vi "CommonVIs_UpdateClassMethods.vi"(1 "ClassPath/LvClassRef":variant, 2 "Methods":string[](array[string]), 4 "AllowPropertyMethod(True)":bool=TRUE, 5 "error in (no error)":errorcluster, 6 "BaseClass":bool, 7 "Don'tShowDialog(False)":bool, 8 "UseVirtualMethods(True)":bool=TRUE) -> (19 "error out":errorcluster)   [LabVIEW 2020]
uses:
  <resource>/Framework/Providers/Open_GDS/ClassProviders/Provider_LvNativeClass/ClassWriterNative_class/ClassWriterNative.lvclass
  <resource>/Framework/Providers/Open_GDS/ClassProviders/Provider_BaseClassInterface/CreateMethodData.ctl
  <resource>/Framework/Providers/Open_GDS/ClassProviders/Provider_EndevoGOOP300/GOOP300_SubVIs/GOOP300_MethodScopeType.ctl
  <resource>/Framework/Providers/Open_GDS/ClassProviders/Provider_LvNativeClass/ClassWriterNative_class/IconDetails.ctl
  <resource>/Framework/Providers/Open_GDS/ClassProviders/Provider_LvNativeClass/ClassWriterNative_class/IconSize.ctl
  <resource>/Framework/Providers/Open_GDS/ClassProviders/Provider_BaseClassInterface/ClassReader_class/ClassReader.lvclass
  <resource>/Framework/Providers/Open_GDS/ClassProviders/Provider_BaseClassInterface/ClassWriter_class/ClassWriter.lvclass
panel:
  out "Creating methods":u8(slide) scale=0.0..100.0
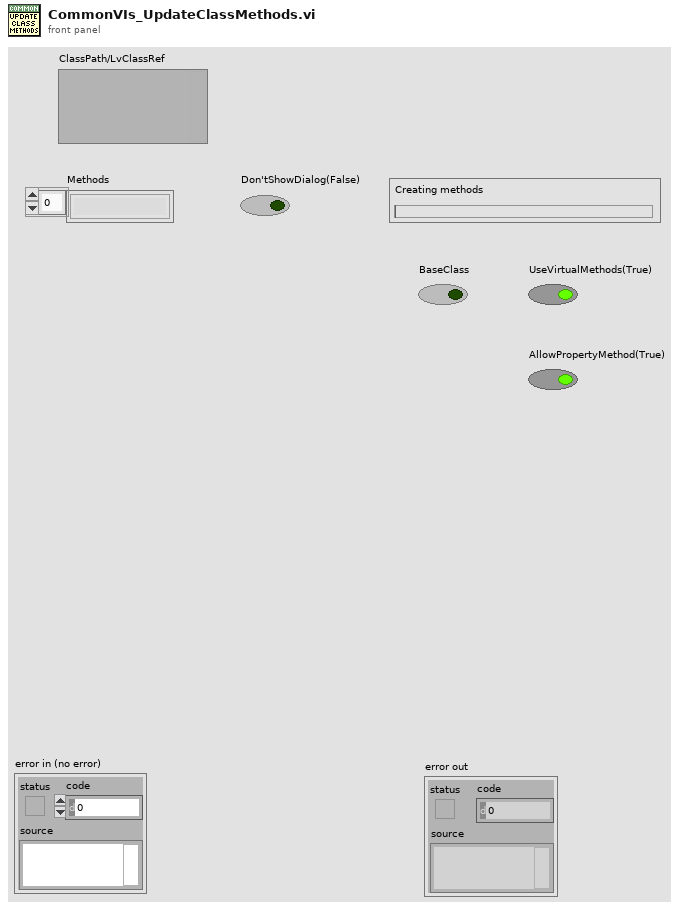
[diagram p1: front panel]
types:
  T1 = cluster{"Methods":cluster{"MethodName":string, "Private":bool, "Virtual":bool, "Reentrant":bool, "Description":string, "Icon Method Name":string, "Protected":bool, "Method Type":enum16{"Get", "Set", "GetProperty", "SetProperty"}, "Attribute":string, "ClassAtt":bool}[], "MethodPaths":path[], "MethodPrivate":bool[], "ClassItemRef":refnum<vi>}
  T2 = cluster{"MethodName":string, "Private":bool, "Virtual":bool, "Reentrant":bool, "Description":string, "Icon Method Name":string, "Protected":bool, "Method Type":enum16{"Get", "Set", "GetProperty", "SetProperty"}, "Attribute":string, "ClassAtt":bool}
  T3 = cluster{"MethodName":string, "Private":bool, "Virtual":bool, "Reentrant":bool, "Description":string, "Icon Method Name":string, "Protected":bool, "Method Type":enum16{"Get", "Set", "GetProperty", "SetProperty"}, "Attribute":string, "ClassAtt":bool}[]
  T4 = enum16{"Get", "Set", "GetProperty", "SetProperty"}
  T5 = typedef "ClassWriter.lvclass/CreateMethodData.ctl" = cluster{"MethodName":string, "RelativeMethodPath":path, "MethodDescription":string, "Scope/Visibility":T6, "MethodTemplateName":string, "IconOut":u8[][], "RelativeProjectClassPath":string, "OpenViAfterCreation":bool, "DynamicDispatchVi":bool, "ExtraCreateParameters":variant, "MustOverride":bool, "MustCallParent":bool, "IconDetails":T7, "AF-Option":variant, "TemplatePath":path}
  T6 = typedef "GOOP300_MethodScopeType.ctl" = enum16{"Use Parent Folder Scope", "Public", "Protected", "Private", "Community"}
  T7 = typedef "ClassWriterNative.lvclass/IconDetails.ctl" = cluster{"IconSize":T8, "ImageRows(32)":i32, "ConnectorPaneHeight":i32[]}
  T8 = typedef "ClassWriterNative.lvclass/IconSize.ctl" = enum16{"Full", "1 c-term high", "2 c-term high", "3 c-term high"}
  T9 = cluster{"AttributeNames":string[], "PropertyNode":bool, "FolderNames":string[]}
  T10 = typedef "ClassTypes_MethodType.ctl" = cluster{"MethodName":string, "Visibility":enum16{"Public", "Private", "Protected"}, "StereoType":string, "Path":path}
  T11 = typedef "CommonVIs_AttributeInfoType.ctl" = cluster{"name":string, "type":T12, "dimension":i32, "typeName":string, "typePath":path, "visibility":T13}
  T12 = typedef "CommonVIs_AttributeDataType.ctl" = enum16{"UINT8", "INT8", "UINT16", "INT16", "UINT32", "INT32", "UINT64", "INT64", "SGL", "DBL", "EXT", "CSG", "CDB", "CXT", "TimeStamp", "STRING", "PATH", "BOOL", "ENUM", "RefNum", "VIRefNum", "LabVIEW Class", "Cluster", "Variant", "TypeDef", "Waveform", "LabVIEW Object", "Other", "void", "Set", "Map"}
  T13 = typedef "CommonVIs_VisibilityType.ctl" = enum16{"Public", "Private", "Protected"}
  T14 = typedef "GDSLvCLass_ClassSettingsType.ctl" = cluster{"ClassProviderName":string, "ClassTemplateUsed":string, "ClassTemplateVersion":string, "ClassDescription":string, "PlugIns":T15[], "ConnectorPanePattern":string}
  T15 = typedef "GDSLvClass_PlugIn.ctl" = cluster{"Type":T16, "ID":string, "Version":string, "Path":path, "Name":string, "Data":variant}
  T16 = typedef "GDSLvClass_PlugInTypes.ctl" = enum16{"DesignPattern", "MethodTypes"}
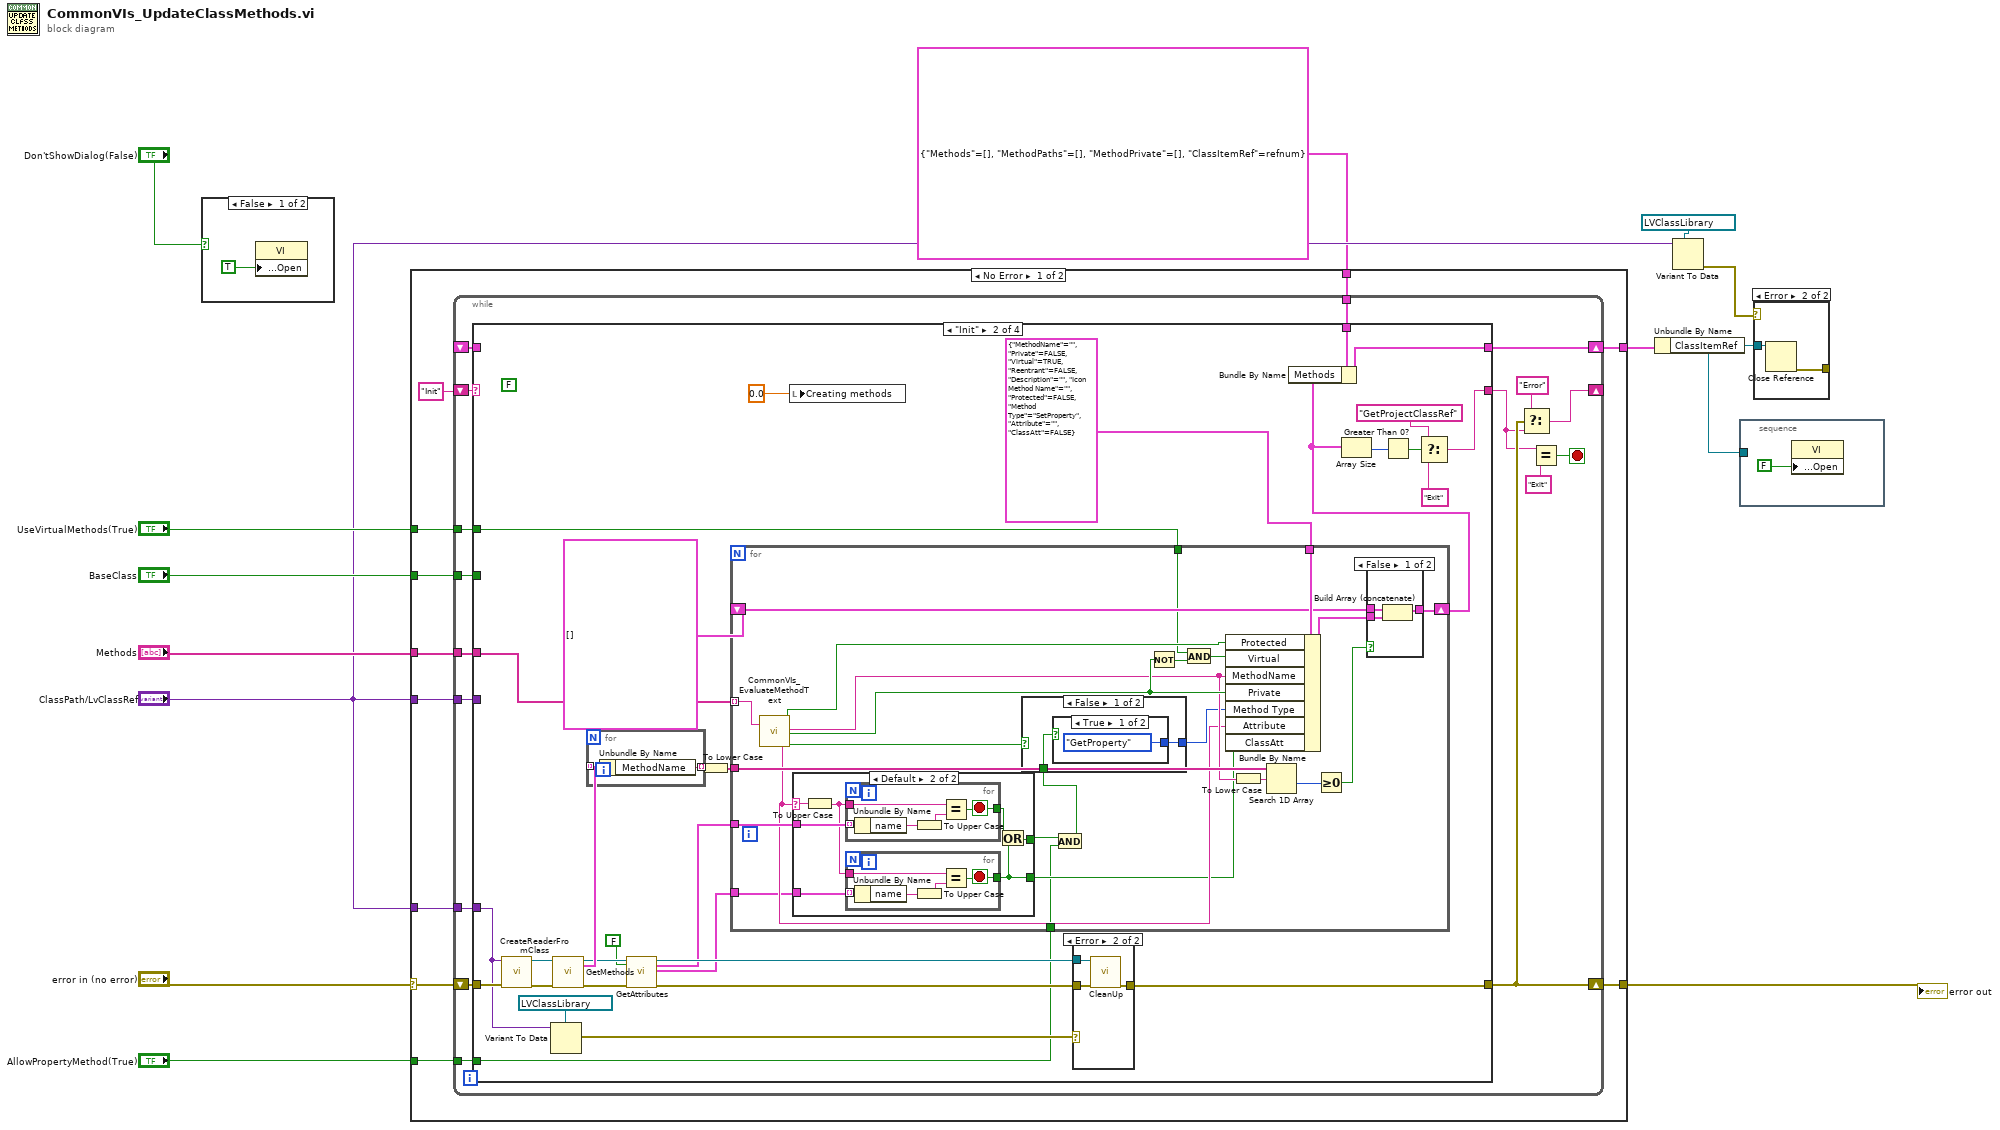
[diagram p0: block diagram]
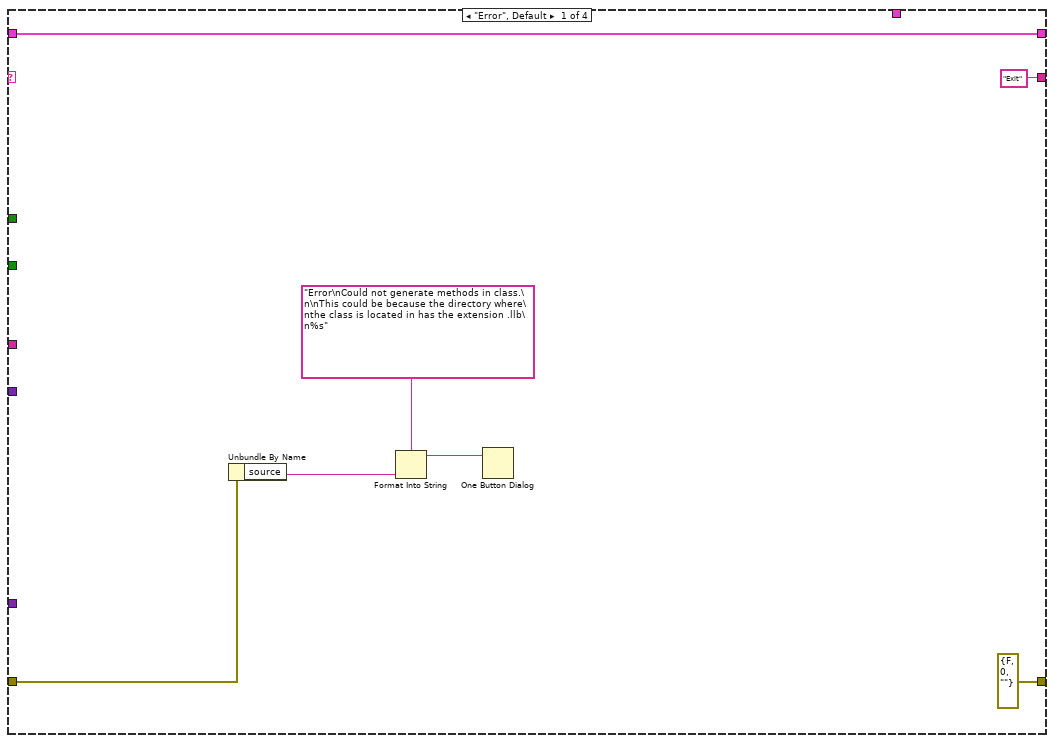
[diagram p4: hidden frame]
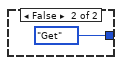
[diagram p7: hidden frame]
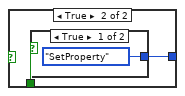
[diagram p8: hidden frame]
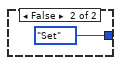
[diagram p9: hidden frame]
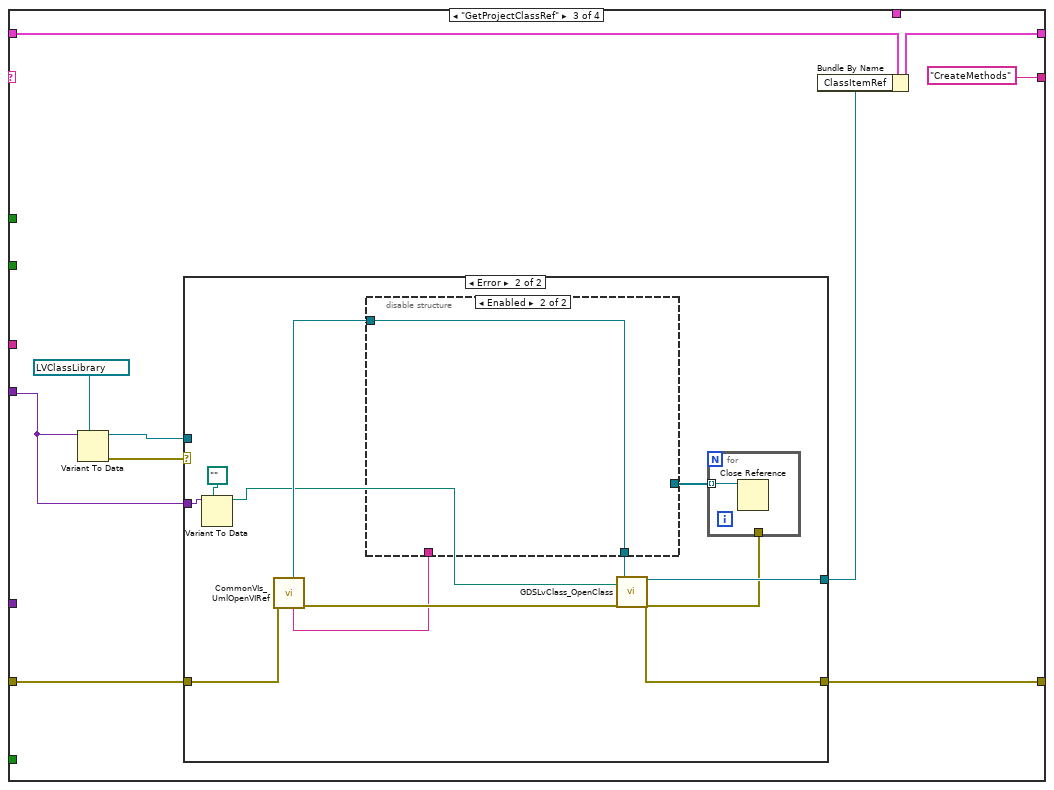
[diagram p11: hidden frame]
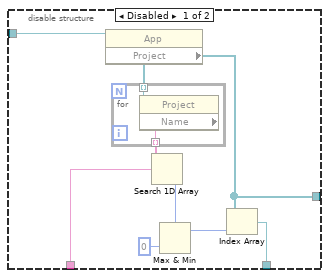
[diagram p13: hidden frame]
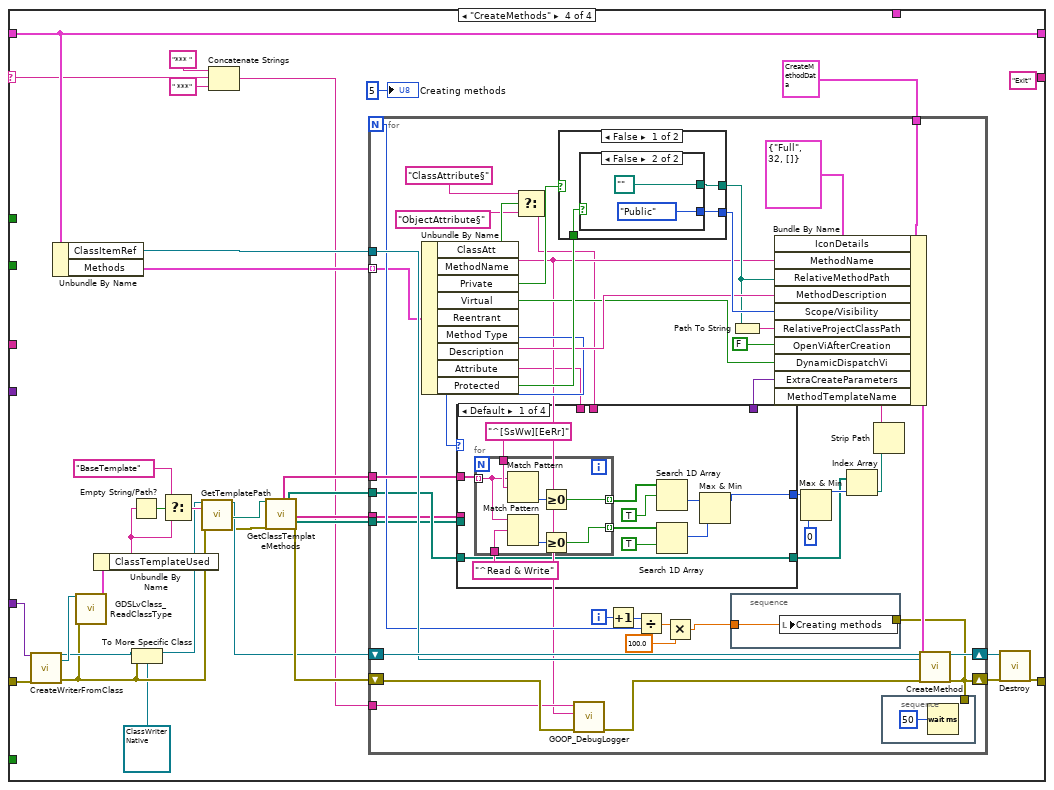
[diagram p14: hidden frame]
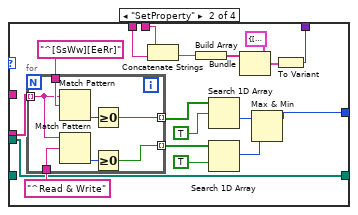
[diagram p15: hidden frame]
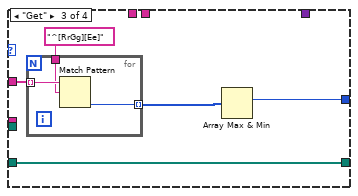
[diagram p16: hidden frame]
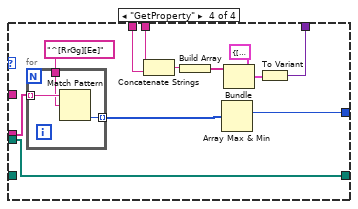
[diagram p17: hidden frame]
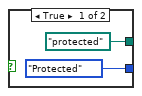
[diagram p18: hidden frame]
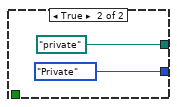
[diagram p19: hidden frame]
diagram:
  n1 = case shown="False" "Don'tShowDialog(False)" {
    frame False {
      n2 = property class="VI"("Front Panel.Open"=TRUE ("Front Panel Window:Open")) -> ()  [unwired: 2 in, 2 out]
    }
    frame True {
    }
  }
  n3 = case shown="No Error" "error in (no error)" {
    selector: "error in (no error)" -> [w25 w327]
    tunnel: [w24 w327] -> w11
    tunnel: "ClassPath/LvClassRef" -> [w22 _]
    tunnel: "Methods" -> [w21 _]
    tunnel: "ClassPath/LvClassRef" -> [w20 _]
    tunnel: [w19 _] -> w10
    tunnel: "BaseClass" -> [w18 _]
    tunnel: "UseVirtualMethods(True)" -> [w17 _]
    tunnel: T1 {"Methods"=[], "MethodPaths"=[], "MethodPrivate"=[], "ClassItemRef"=refnum} -> [w16 _]
    tunnel: "AllowPropertyMethod(True)" -> [w15 _]
    frame No Error {
      n4 = while {
        shift-right: [w35] -> w24
        shift-left: w25 -> [w41]
        shift-right: [w36] -> _
        shift-left: "Init" -> [w42]
        tunnel: w22 -> [w40]
        shift-right: [w39] -> w19
        shift-left: _ -> [w38]
        tunnel: w21 -> [w31]
        tunnel: w20 -> [w30]
        tunnel: w18 -> [w29]
        tunnel: w17 -> [w28]
        tunnel: w16 -> [w27]
        tunnel: w15 -> [w26]
        stop <- w32 stop-if-true
        n5 = case shown="\"Init\"" w42 {
          selector: w42 -> [_ _ _ w178]
          tunnel: w41 -> [w46 w62 w146 w204]
          tunnel: w40 -> [_ w60 _ w186]
          tunnel: ["Exit" ("y") w72 "CreateMethods" ("y") "Exit" ("y")] -> w34
          tunnel: [w48 w80 w147 w183] -> w39
          tunnel: [errorcluster {"status"=FALSE, "code"=0, "source"=""} ("error out") w69 w144 w184] -> w35
          tunnel: w38 -> [w48 _ w148 w183]
          tunnel: w31 -> [_ w79 _ _]
          tunnel: w30 -> [_ _ w142 _]
          tunnel: w29 -> [_ _ _ _]
          tunnel: w28 -> [_ w64 _ _]
          tunnel: w27 -> [_ w53 _ _]
          tunnel: w26 -> [_ w50 _ _]
          frame "Error", Default {
            n6 = Unbundle By Name(w46) -> ("source"=w45:string)
            n7 = Format Into String(format string="Error\nCould not generate methods in class.\n\nThis could be because the directory where\nthe class is located in has the extension .llb\n%s" ("message"), w45) -> (resulting string=w44:string)  [unwired: 2 in, 1 out]
            n8 = One Button Dialog(message=w44) -> ()  [unwired: 2 out]
          }
          frame "Init" {
            (unwired) FALSE
            n9 = call <resource>:"CreateReaderFromClass.vi"("ClassPath/LvClassRef"=w60, "error in"=w62) -> ("ClassReader"=w71:refnum<class "ClassReader.lvclass">, "error out"=w70:errorcluster)  [unwired: 16 out]
            n10 = Variant To Data(type=refnum<vi> refnum ("LVClass.Open"), Variant=w60) -> (error out=w59:errorcluster)  [unwired: 1 in, 1 out]
            n11 = call-dynamic "GetMethods.vi"("ClassReader in"=w71, "error in (no error)"=w70) -> ("ClassReader out"=w58:refnum<class "ClassReader.lvclass">, "Methods"=w68:T10[], "error out"=w57:errorcluster)  [unwired: 15 out]
            n12 = for {
              tunnel: w68 -> [w86] mode=indexing
              tunnel: [w85] -> w67 mode=indexing
              n13 = Unbundle By Name(w86) -> ("MethodName"=w85:string)
            }
            n14 = call-dynamic "GetAttributes.vi"("ClassReader in"=w58, "OnlyGetReference"=FALSE, "error in (no error)"=w57) -> ("ClassReader out"=w56:refnum<class "ClassReader.lvclass">, "ObjectAttributes"=w52:T11[], "ClassAttributes"=w51:T11[], "error out"=w55:errorcluster)  [unwired: 11 in, 2 out]
            n15 = To Lower Case(string=w67) -> (all lower case string=w66:string[])
            n16 = for {
              tunnel: w79 -> [w97] mode=indexing
              tunnel: T2 {"MethodName"="", "Private"=FALSE, "Virtual"=TRUE, "Reentrant"=FALSE, "Description"="", "Icon Method Name"="", "Protected"=FALSE, "Method Type"=enum."SetProperty", "Attribute"="", "ClassAtt"=FALSE} ("element") -> [w110]
              shift-right: [w109] -> w77
              shift-left: T3 [] -> [w108]
              tunnel: w66 -> [w105]
              tunnel: w64 -> [w98]
              tunnel: w52 -> [w93]
              tunnel: w51 -> [w91]
              tunnel: w50 -> [w89]
              n17 = call <resource>:"CommonVIs_EvaluateMethodText.vi"("String"=w97) -> ("MethodAttributeName"=w92:string, "Protected"=w102:bool, "MethodName"=w96:string, "Private"=w100:bool, "SetMethod"=w95:bool)  [unwired: 1 in, 13 out]
              n18 = case shown="Default" w92 {
                selector: w92 -> [_ w116]
                tunnel: w93 -> [_ w117]
                tunnel: [_ w112] -> w87
                tunnel: w91 -> [_ w114]
                tunnel: [_ w111] -> w90
                frame "" {
                }
                frame Default {
                  n19 = To Upper Case(1:w116) -> (0:w115:string)
                  n20 = for {
                    tunnel: w117 -> [w127] mode=indexing
                    tunnel: w115 -> [w124]
                    tunnel: [w123] -> w113
                    stop <- w123 stop-if-true
                    n21 = Unbundle By Name(w127) -> ("name"=w126:string)
                    n22 = To Upper Case(1:w126) -> (0:w125:string)
                    n23 = Equal?(x=w124, y=w125) -> (x = y?=w123:bool)
                  }
                  n24 = for {
                    tunnel: w114 -> [w122] mode=indexing
                    tunnel: w115 -> [w119]
                    tunnel: [w118] -> w111
                    stop <- w118 stop-if-true
                    n25 = Unbundle By Name(w122) -> ("name"=w121:string)
                    n26 = To Upper Case(1:w121) -> (0:w120:string)
                    n27 = Equal?(x=w119, y=w120) -> (x = y?=w118:bool)
                  }
                  n28 = Or(x=w113, y=w111) -> (x .or. y?=w112:bool)
                }
              }
              n29 = And(x=w87, y=w89) -> (x .and. y?=w88:bool)
              n30 = case shown="False" w95 {
                tunnel: [w129 w133] -> w94
                tunnel: w88 -> [w128 w132]
                frame False {
                  n31 = case shown="True" w128 {
                    tunnel: [T4."GetProperty" ("Method Type") T4."Get" ("Method Type")] -> w129
                    frame True {
                    }
                    frame False {
                    }
                  }
                }
                frame True {
                  n32 = case shown="True" w132 {
                    tunnel: [T4."SetProperty" ("Method Type") T4."Set" ("Method Type")] -> w133
                    frame True {
                    }
                    frame False {
                    }
                  }
                }
              }
              n33 = Not(x=w100) -> (.not. x?=w101:bool)
              n34 = And(x=w98, y=w101) -> (x .and. y?=w99:bool)
              n35 = Bundle By Name(cluster=w110, "Protected"=w102, "Virtual"=w99, "MethodName"=w96, "Private"=w100, "Method Type"=w94, "Attribute"=w92, "ClassAtt"=w90) -> (w107:T2)
              n36 = To Lower Case(string=w96) -> (all lower case string=w106:string)
              n37 = Search 1D Array(1D array=w105, element=w106) -> (index of element=w104:i32)  [unwired: 1 out]
              n38 = Greater Or Equal To 0?(x=w104) -> (x >= 0?=w103:bool)
              n39 = case shown="False" w103 {
                tunnel: [w138 w139] -> w109
                tunnel: w108 -> [w137 w139]
                tunnel: w107 -> [w136 _]
                frame False {
                  n40 = Build Array (concatenate)(w137, w136) -> (w138:T3)
                }
                frame True {
                }
              }
            }
            n41 = local write "Creating methods"(0.0 ("Methods (%)")) -> ()
            n42 = case shown="Error" w59 {
              tunnel: w55 -> [w81 w84]
              tunnel: w56 -> [_ w83]
              tunnel: [w81 w82] -> w69
              frame No Error {
              }
              frame Error {
                n43 = call-dynamic "CleanUp.vi"("reference in"=w83, "error in (no error)"=w84) -> ("error out"=w82:errorcluster)  [unwired: 17 out]
              }
            }
            n44 = Bundle By Name(cluster=w53, "Methods"=w77) -> (w80:T1)
            n45 = Array Size(array=w77) -> (size(s)=w76:i32)
            n46 = Greater Than 0?(x=w76) -> (x > 0?=w75:bool)
            n47 = Select(t="GetProjectClassRef" ("y"), s=w75, f="Exit" ("y")) -> (s? t:f=w72:string)
          }
          frame "GetProjectClassRef" {
            n48 = Variant To Data(type=refnum<vi> refnum ("LVClass.Open"), Variant=w142) -> (data=w140:refnum<vi>, error out=w141:errorcluster)  [unwired: 1 in]
            n49 = case shown="Error" w141 {
              tunnel: w146 -> [w150 w158]
              tunnel: [w151 w157] -> w145
              tunnel: [w150 w152] -> w144
              tunnel: w142 -> [_ w155]
              tunnel: w140 -> [w151 _]
              frame No Error {
              }
              frame Error {
                n50 = Variant To Data(type=path "", Variant=w155) -> (data=w154:path)  [unwired: 1 in, 1 out]
                n51 = call <resource>:"CommonVIs_UmlOpenVIRef.vi"("error in"=w158) -> ("error out"=w162:errorcluster, "ProjectNameOut"=w160:string, "AppRefOut"=w161:refnum<vi>)  [unwired: 3 in, 5 out]
                n52 = disable-structure shown="Enabled" {
                  disable-tunnel: w161 -> [w166 w173]
                  disable-tunnel: w160 -> [w165 _]
                  disable-tunnel: [w164 w173] -> w159
                  disable-tunnel: [w163 _] -> w153
                  frame Disabled {
                    n53 = property class="App"(reference=w166) -> ("Project"=w163:refnum<vi>[])  [unwired: 1 in, 2 out]
                    n54 = for {
                      tunnel: w163 -> [w172] mode=indexing
                      tunnel: [w171] -> w170 mode=indexing
                      n55 = property class="Project"(reference=w172) -> ("Name"=w171:string)  [unwired: 1 in, 2 out]
                    }
                    n56 = Search 1D Array(1D array=w170, element=w165) -> (index of element=w169:i32)  [unwired: 1 out]
                    n57 = Max & Min(x=w169, y=0) -> (max(x,y)=w167:i32)  [unwired: 1 out]
                    n58 = Index Array(array=w163, index=w167) -> (element=w164:refnum<vi>)
                  }
                  frame Enabled {
                  }
                }
                n59 = call <resource>:"GDSLvClass_OpenClass.vi"("ClassToOpen"=w154, "error in (no error)"=w162, "Project/ApplicationRef(If empty, currect active project will be used)"=w159) -> ("LVClass.Open"=w157:refnum<vi>, "error out"=w152:errorcluster)  [unwired: 15 out]
                n60 = for {
                  tunnel: w153 -> [w174] mode=indexing
                  tunnel: w152 -> [_]
                  n61 = Close Reference(reference=w174) -> ()  [unwired: 1 in, 1 out]
                }
              }
            }
            n62 = Bundle By Name(cluster=w148, "ClassItemRef"=w145) -> (w147:T1)
          }
          frame "CreateMethods" {
            n63 = call <resource>:"CreateWriterFromClass.vi"("ClassPath/LvClassRef"=w186, "error in"=w204) -> ("ClassWriter"=w192:refnum<class "ClassWriter.lvclass">, "LVClassRef"=w197:refnum<vi>, "error out"=w191:errorcluster)  [unwired: 15 out]
            n64 = Unbundle By Name(w183) -> ("ClassItemRef"=w203:refnum<vi>, "Methods"=w205:T3)
            n65 = call <resource>:"GDSLvClass_ReadClassType.vi"("Class Refnum In"=w197, "error in (no error)"=w191) -> ("ClassSettings"=w200:T14)  [unwired: 17 out]
            n66 = Unbundle By Name(w200) -> ("ClassTemplateUsed"=w199:string)
            n67 = Empty String/Path?(string/path=w199) -> (empty?=w202:bool)
            n68 = To More Specific Class(target class=refnum<class "ClassWriterNative.lvclass"> refnum ("reference in"), reference=w192, error in=w191) -> (specific class reference=w189:refnum<class "ClassWriterNative.lvclass">)  [unwired: 1 out]
            n69 = Select(t="BaseTemplate", s=w202, f=w199) -> (s? t:f=w198:string)
            n70 = call-dynamic "GetTemplatePath.vi"("reference in"=w189, "ClassTemplateSubDirectory"=w198, "error in (no error)"=w191) -> ("reference out"=w188:refnum<class "ClassWriterNative.lvclass">, "MethodTemplatePathOut"=w196:path, "error out"=w182:errorcluster)  [unwired: 14 out]
            n71 = Concatenate Strings("*** " ("string"), w178, " ***" ("string")) -> (w176:string)
            n72 = call <resource>:"GetClassTemplateMethods.vi"("MethodTemplatePath"=w196, "error in"=w182) -> ("NormalMethodNames"=w194:string[], "NormalMethodPaths"=w193:path[], "PropertyMethodNames"=w181:string[], "PropertyMethodPaths"=w180:path[], "error out"=w195:errorcluster)  [unwired: 13 out]
            n73 = for {
              N -> [w232]
              tunnel: w205 -> [w210] mode=indexing
              tunnel: w203 -> [w248]
              shift-right: [w208] -> w184
              shift-left: w195 -> [w224]
              tunnel: w194 -> [w242]
              tunnel: w193 -> [w220]
              shift-right: [w227] -> w185
              shift-left: w188 -> [w249]
              tunnel: w176 -> [w222]
              tunnel: w181 -> [w218]
              tunnel: w180 -> [w217]
              tunnel: T5 {"MethodName"="", "RelativeMethodPath"=path "", "MethodDescription"="", "Scope/Visibility"=enum."Use Parent Folder Scope", "MethodTemplateName"="", "IconOut"=[], "RelativeProjectClassPath"="", "OpenViAfterCreation"=FALSE, "DynamicDispatchVi"=FALSE, "ExtraCreateParameters"=variant, "MustOverride"=FALSE, "MustCallParent"=FALSE, "IconDetails"={"IconSize"=enum."Full", "ImageRows(32)"=0, "ConnectorPaneHeight"=[]}, "AF-Option"=variant, "TemplatePath"=path ""} ("CreateMethodData") -> [w209]
              i -> [w233]
              n74 = Unbundle By Name(w210) -> ("ClassAtt"=w214:bool, "MethodName"=w221:string, "Private"=w246:bool, "Virtual"=w236:bool, "Method Type"=w225:T4, "Description"=w243:string, "Attribute"=w215:string, "Protected"=w244:bool)  [unwired: 1 out]
              n75 = Select(t="ClassAttribute§" ("string"), s=w214, f="ObjectAttribute§" ("string")) -> (s? t:f=w211:string)
              n76 = case shown="Default" w225 {
                tunnel: w242 -> [w261 _ w298 _]
                tunnel: [w252 w278 w296 w312] -> w241
                tunnel: w220 -> [w251 _ w294 _]
                tunnel: [w251 w276 w294 w309] -> w219
                tunnel: w218 -> [_ w277 _ w310]
                tunnel: w217 -> [_ w276 _ w309]
                tunnel: w215 -> [_ w275 _ w308]
                tunnel: [_ w269 _ w302] -> w216
                tunnel: w211 -> [_ w274 _ w307]
                frame Default {
                  n77 = for {
                    tunnel: w261 -> [w264] mode=indexing
                    tunnel: "^[SsWw][EeRr]" -> [w268]
                    tunnel: [w266] -> w256 mode=indexing
                    tunnel: "^Read & Write" -> [w263]
                    tunnel: [w262] -> w258 mode=indexing
                    n78 = Match Pattern(string=w264, regular expression=w268) -> (offset past match=w267:i32)  [unwired: 4 out]
                    n79 = Match Pattern(string=w264, regular expression=w263) -> (offset past match=w265:i32)  [unwired: 4 out]
                    n80 = Greater Or Equal To 0?(x=w267) -> (x >= 0?=w266:bool)
                    n81 = Greater Or Equal To 0?(x=w265) -> (x >= 0?=w262:bool)
                  }
                  n82 = Search 1D Array(1D array=w256, element=TRUE) -> (index of element=w254:i32)  [unwired: 1 out]
                  n83 = Search 1D Array(1D array=w258, element=TRUE) -> (index of element=w253:i32)  [unwired: 1 out]
                  n84 = Max & Min(x=w254, y=w253) -> (max(x,y)=w252:i32)  [unwired: 1 out]
                }
                frame "SetProperty" {
                  n85 = for {
                    tunnel: w277 -> [w289] mode=indexing
                    tunnel: "^[SsWw][EeRr]" -> [w293]
                    tunnel: [w291] -> w282 mode=indexing
                    tunnel: "^Read & Write" -> [w288]
                    tunnel: [w287] -> w284 mode=indexing
                    n86 = Match Pattern(string=w289, regular expression=w293) -> (offset past match=w292:i32)  [unwired: 4 out]
                    n87 = Match Pattern(string=w289, regular expression=w288) -> (offset past match=w290:i32)  [unwired: 4 out]
                    n88 = Greater Or Equal To 0?(x=w292) -> (x >= 0?=w291:bool)
                    n89 = Greater Or Equal To 0?(x=w290) -> (x >= 0?=w287:bool)
                  }
                  n90 = Concatenate Strings(w274, w275) -> (w270:string)
                  n91 = Build Array(w270) -> (w272:string[])
                  n92 = Search 1D Array(1D array=w282, element=TRUE) -> (index of element=w280:i32)  [unwired: 1 out]
                  n93 = Search 1D Array(1D array=w284, element=TRUE) -> (index of element=w279:i32)  [unwired: 1 out]
                  n94 = Bundle(cluster=T9 {"AttributeNames"=[], "PropertyNode"=FALSE, "FolderNames"=[]}, "AttributeNames"=w272) -> (w273:T9)  [unwired: 2 in]
                  n95 = Max & Min(x=w280, y=w279) -> (max(x,y)=w278:i32)  [unwired: 1 out]
                  n96 = To Variant(anything=w273) -> (Variant=w269:variant)
                }
                frame "Get" {
                  n97 = for {
                    tunnel: w298 -> [w301] mode=indexing
                    tunnel: "^[RrGg][Ee]" -> [w300]
                    tunnel: [w299] -> w297 mode=indexing
                    n98 = Match Pattern(string=w301, regular expression=w300) -> (offset past match=w299:i32)  [unwired: 4 out]
                  }
                  n99 = Array Max & Min(array=w297) -> (max index (indices)=w296:i32)  [unwired: 3 out]
                }
                frame "GetProperty" {
                  n100 = for {
                    tunnel: w310 -> [w316] mode=indexing
                    tunnel: "^[RrGg][Ee]" -> [w315]
                    tunnel: [w314] -> w313 mode=indexing
                    n101 = Match Pattern(string=w316, regular expression=w315) -> (offset past match=w314:i32)  [unwired: 4 out]
                  }
                  n102 = Concatenate Strings(w307, w308) -> (w303:string)
                  n103 = Build Array(w303) -> (w305:string[])
                  n104 = Array Max & Min(array=w313) -> (max index (indices)=w312:i32)  [unwired: 3 out]
                  n105 = Bundle(cluster=T9 {"AttributeNames"=[], "PropertyNode"=FALSE, "FolderNames"=[]}, "AttributeNames"=w305) -> (w306:T9)  [unwired: 2 in]
                  n106 = To Variant(anything=w306) -> (Variant=w302:variant)
                }
              }
              n107 = case shown="False" w246 {
                tunnel: [w318 path "private"] -> w234
                tunnel: [w319 GOOP300_MethodScopeType."Private" ("Scope/Visibility")] -> w245
                tunnel: w244 -> [w320 _]
                frame False {
                  n108 = case shown="False" w320 {
                    tunnel: [path "protected" path ""] -> w318
                    tunnel: [GOOP300_MethodScopeType."Protected" ("Scope/Visibility") GOOP300_MethodScopeType."Public" ("Scope/Visibility")] -> w319
                    frame True {
                    }
                    frame False {
                    }
                  }
                }
                frame True {
                }
              }
              n109 = call <resource>:"GOOP_DebugLogger.vi"("error in (no error)"=w224, "Data"=w221, "State"=w222) -> ("error out"=w223:errorcluster)  [unwired: 6 in, 2 out]
              n110 = Increment(x=w233) -> (x+1=w231:i32)
              n111 = Divide(x=w231, y=w232) -> (x/y=w230:dbl)
              n112 = Multiply(x=w230, y=100.0) -> (x*y=w228:dbl)
              n113 = Path To String(path=w234) -> (string=w235:string)
              n114 = Max & Min(x=w241, y=0) -> (max(x,y)=w239:i32)  [unwired: 1 out]
              n115 = Index Array(array=w219, index=w239) -> (element=w238:path)
              n116 = Strip Path(path=w238) -> (name=w226:string)  [unwired: 1 out]
              n117 = Bundle By Name(cluster=w209, "IconDetails"=T7 {"IconSize"=enum."Full", "ImageRows(32)"=32, "ConnectorPaneHeight"=[]}, "MethodName"=w221, "RelativeMethodPath"=w234, "MethodDescription"=w243, "Scope/Visibility"=w245, "RelativeProjectClassPath"=w235, "OpenViAfterCreation"=FALSE, "DynamicDispatchVi"=w236, "ExtraCreateParameters"=w216, "MethodTemplateName"=w226) -> (w247:T5)
              n118 = call-dynamic "CreateMethod.vi"("ClassWriterNative.lvclass"=w249, "ClassItemRefIn"=w248, "CreateMethodData"=w247, "error in (no error)"=w223) -> ("ClassWriterNative.lvclass 2"=w227:refnum<class "ClassWriterNative.lvclass">, "error out"=w208:errorcluster)  [unwired: 14 out]
              n119 = stacked-sequence {
                tunnel: w208 -> [_]
                tunnel: w228 -> [w317]
                frame #0 {
                  n120 = local write "Creating methods"(w317) -> ()
                }
              }
              n121 = stacked-sequence {
                tunnel: w208 -> [_]
                frame #0 {
                  n122 = Wait (ms)(milliseconds to wait=u32 50) -> ()  [unwired: 1 out]
                }
              }
            }
            n123 = call-dynamic "Destroy.vi"("ClassWriterNative"=w185, "error in (no error)"=w184) -> ()  [unwired: 18 out]
            "Creating methods" <- u8 5 ("Creating methods")
          }
        }
        n124 = Select(t="Error", s=w35, f=w34) -> (s? t:f=w36:string)
        n125 = Equal?(x=w34, y="Exit") -> (x = y?=w32:bool)
      }
    }
    frame Error {
    }
  }
  "error out" <- w11
  n126 = Unbundle By Name(w10) -> ("ClassItemRef"=w3:refnum<vi>)
  n127 = Variant To Data(type=refnum<vi> refnum ("LVClass.Open"), Variant="ClassPath/LvClassRef") -> (error out=w5:errorcluster)  [unwired: 1 in, 1 out]
  n128 = stacked-sequence {
    tunnel: w3 -> [_]
    frame #0 {
      n129 = property class="VI"("Front Panel.Open"=FALSE ("Front Panel Window:Open")) -> ()  [unwired: 2 in, 2 out]
    }
  }
  n130 = case shown="Error" w5 {
    tunnel: w3 -> [_ w330]
    tunnel: [_ w329] -> _
    frame No Error {
    }
    frame Error {
      n131 = Close Reference(reference=w330) -> (error out=w329:errorcluster)  [unwired: 1 in]
    }
  }
